vi "Write File.vi"(8 "error in (no error)":errorcluster, 11 "Data.HDF5 in":refnum<class "Data.HDF5.lvclass">) -> (0 "error out":errorcluster, 3 "Data.HDF5 out":refnum<class "Data.HDF5.lvclass">)   [LabVIEW 2016, in "Data.HDF5.lvclass"]
uses:
  Data.HDF5.lvclass
  Data/Data.lvclass
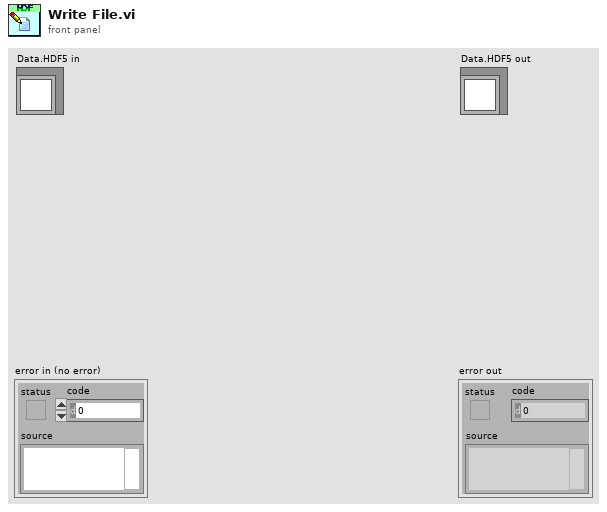
[diagram p1: front panel]
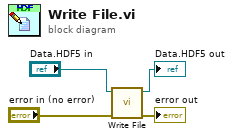
[diagram p0: block diagram]
diagram:
  n1 = call-parent "Write File.vi"("error in (no error)"="error in (no error)", "Data in"="Data.HDF5 in") -> ("error out"=→"error out":errorcluster, "Data out"=→"Data.HDF5 out":refnum<class "Data.HDF5.lvclass">)  [unwired: 8 in]
